vi "final.vi"() -> ()   [LabVIEW 2018]
uses:
  <vilib>/DAQmx/read.llb/DAQmx Read (Analog DBL 1Chan 1Samp).vi
  <vilib>/DAQmx/create/channels.llb/DAQmx Create Channel (AI-Voltage-Basic).vi
  <vilib>/DAQmx/miscellaneous.llb/DAQmx Fill In Error Info.vi
  <vilib>/Utility/file.llb/Write Delimited Spreadsheet (DBL).vi
  <vilib>/Waveform/WDTOps.llb/WDT Waveform to XY Pairs DBL.vi
  <instrlib>/Agilent 34405/Agilent 34405.lvlib
panel:
  in  "VISA":refnum<visa-resource-name>
  out "Voltage versus Time":dbl(graph)
  out "Current Versus time":dbl(graph)
  out "PWM Graph":waveform(dbl)(graph)
  in  "stop":bool
  in  "file path (dialog if empty)":path
  in  "Ahmeter":refnum<visa-resource-name>
  in  "Counter-clockwise":bool
  in  "Clockwise Rotation":bool
  in  "Nucleo":refnum<visa-resource-name>
  in  "Motor speed (In duty cycle %)":u8(knob) max=100 scale=0.0..100.0
  # "Probe Attenuation MUST BE SET TO X10"
  # "Notes on Controling the direction:\n\nLeaving both buttons off will set the motor to coast\nOnly turning clockwise on will set the motor to turn clockwise\nOnly turning counter-clockwise on will set the motor to turn counter clock-wise\nTurning both on will set the motor to BREAK"
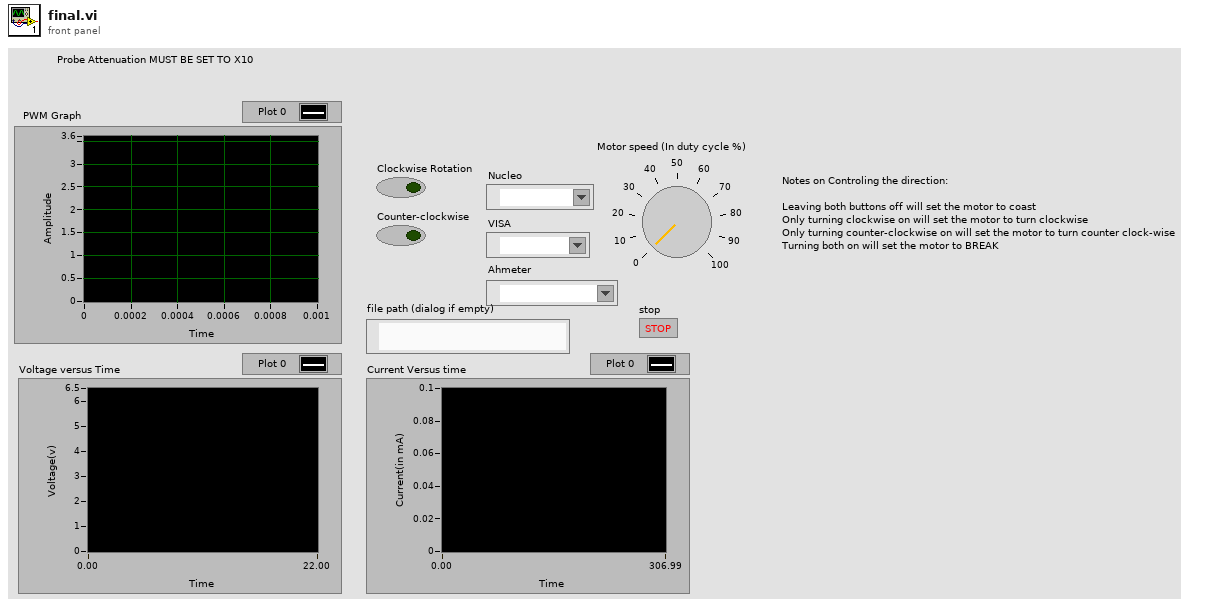
[diagram p1: front panel]
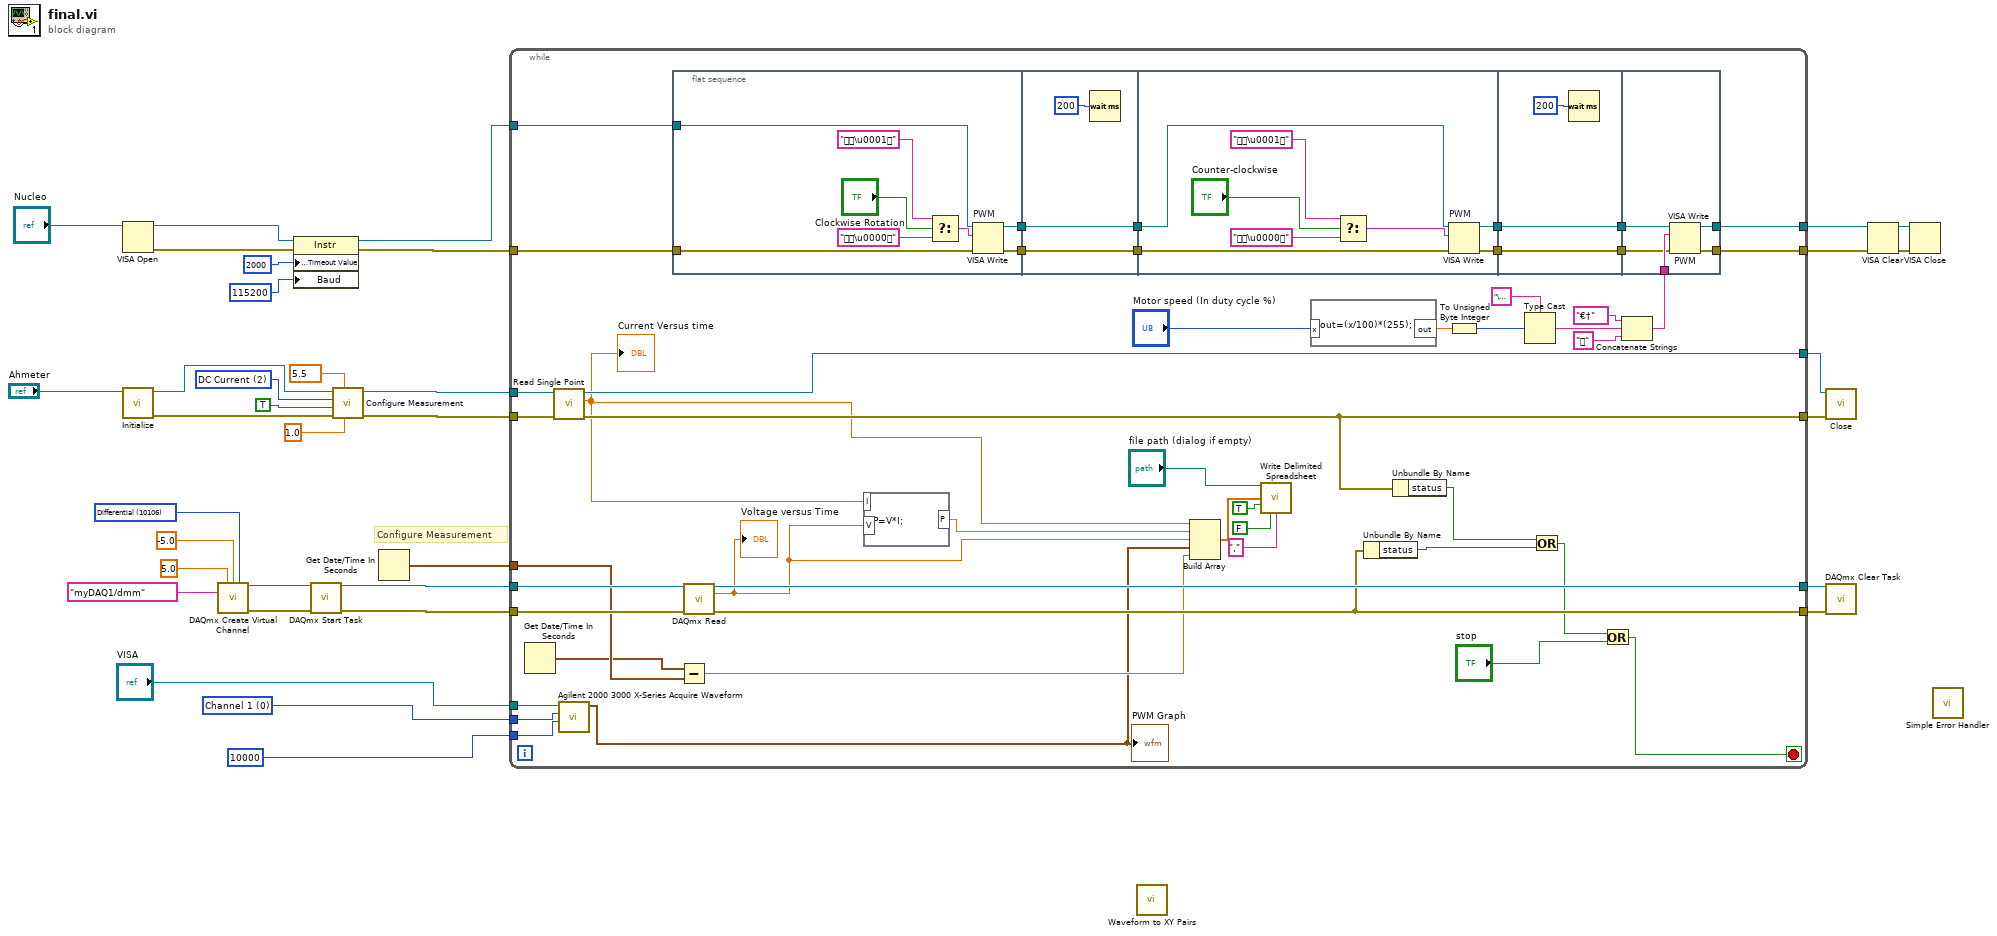
[diagram p0: block diagram]
diagram:
  w2 = 0 items=["Channel 1"=0, "Channel 2"=1, "Channel 3"=2, "Channel 4"=3, "Digital Bus Low"=9, "Digital Bus High"=10] ("Auto Scale Source (0: Channel 1)")
  w11 = 5.5 items=["3.5"=3.5, "4.5"=4.5, "5.5"=5.5] ("Manual Resolution (5.5 Digits)")
  w9 = 2 items=["DC Volts", "AC Volts", "DC Current", "AC Current", "2-Wire Resistance", "Frequency", "Temperature", "Capacitance", "Continuity", "Diode", "4-Wire Resistance", "2nd DC Volts", "2nd AC Volts", "2nd DC Current", "2nd AC Current", "2nd Frequency"] ("Function (0: DC Volts)")
  w22 = 10106 items=["Default"=-1, "RSE"=10083, "NRSE"=10078, "Differential"=10106, "Pseudodifferential"=12529] ("input terminal configuration")
  # "Configure Measurement"
  n1 = VISA Open(VISA resource name="Nucleo") -> (VISA resource name=w33:refnum<visa-resource-name>, error out=w36:errorcluster)  [unwired: 4 in]
  n2 = call <instrlib>:"Initialize.vi"("VISA resource name"="Ahmeter") -> ("error out"=w13:errorcluster, "VISA resource name out"=w14:refnum<visa-resource-name>)  [unwired: 3 in, 6 out]
  n3 = call-poly <vilib>:"DAQmx Create Virtual Channel.vi"("maximum value"=5.0, "minimum value"=-5.0, "input terminal configuration"=w22, "physical channels"=tag "myDAQ1/dmm") -> ("task out"=w27:refnum<k21>, "error out"=w26:errorcluster)  [unwired: 10 in]
  n4 = property class="Instr"(reference=w33, error in=w36, "General Settings:Timeout Value"=u32 2000, "Baud"=u32 115200 ("Serial Settings:Baud Rate")) -> (reference out=w29:refnum<visa-resource-name>, error out=w28:errorcluster)
  n5 = call <vilib>:"DAQmx Start Task.vi"("task/channels in"=w27, "error in"=w26) -> ("task out"=w19:refnum<k21>, "error out"=w18:errorcluster)  [unwired: 12 in]
  n6 = call <instrlib>:"Configure Measurement.vi"("Manual Range (1)"=1.0, "Manual Resolution (5.5 Digits)"=w11, "error in (no error)"=w13, "Enable Auto Range (T:Enable)"=TRUE, "Function (0: DC Volts)"=w9, "VISA resource name"=w14) -> ("error out"=w8:errorcluster, "VISA resource name out"=w7:refnum<visa-resource-name>)  [unwired: 4 out]
  n7 = Get Date/Time In Seconds() -> (seconds since 1Jan1904=w4:timestamp)
  n8 = while {
    tunnel: w29 -> [w84]
    tunnel: w28 -> [w83]
    tunnel: [w56] -> w21
    tunnel: [w50] -> w20
    tunnel: w19 -> [w63]
    tunnel: w18 -> [w62]
    tunnel: [w70] -> w17
    tunnel: [w69] -> w16
    tunnel: w8 -> [w68]
    tunnel: w7 -> [w67]
    tunnel: [w52] -> w6
    tunnel: [w66] -> w5
    tunnel: w4 -> [w53]
    tunnel: "VISA" -> [w40]
    tunnel: w2 -> [w39]
    tunnel: u32 10000 ("Maximum Time (10000 ms)") -> [w38]
    stop <- w46 stop-if-true
    n9 = Get Date/Time In Seconds() -> (seconds since 1Jan1904=w45:timestamp)
    n10 = call <instrlib>:"Read Single Point.vi"("error in (no error)"=w68, "VISA resource name"=w67) -> ("error out"=w52:errorcluster, "Measurement"=w42:dbl, "VISA resource name out"=w66:refnum<visa-resource-name>)  [unwired: 7 out]
    "Current Versus time" <- w42
    n11 = call "Agilent 2000 3000 X-Series Acquire Waveform.vi"("Maximum Time (10000 ms)"=w38, "Auto Scale Source (0: Channel 1)"=w39, "VISA resource name"=w40) -> ("Waveform Data"=w37:waveform(dbl))  [unwired: 8 in]
    "PWM Graph" <- w37
    n12 = flat-sequence {
      tunnel: [w90] -> w78
      tunnel: [w89] -> w77
      tunnel: w84 -> [w92]
      tunnel: w83 -> [w91]
      tunnel: w78 -> [w95]
      tunnel: w77 -> [w94]
      tunnel: [w95] -> w76
      tunnel: [w94] -> w75
      tunnel: w76 -> [w98]
      tunnel: w75 -> [w99]
      tunnel: [w97] -> w65
      tunnel: [w96] -> w64
      tunnel: w65 -> [w104]
      tunnel: w64 -> [w105]
      tunnel: [w105] -> w61
      tunnel: [w104] -> w60
      tunnel: w71 -> [w111]
      tunnel: [w110] -> w70
      tunnel: [w109] -> w69
      tunnel: w61 -> [w108]
      tunnel: w60 -> [w107]
      frame #0 {
        n13 = Select(t="\u0001" ("write buffer"), s="Clockwise Rotation", f="\u0000" ("write buffer")) -> (s? t:f=w85:string)
        n14 = VISA Write "PWM"(VISA resource name=w92, write buffer=w85, error in (no error)=w91) -> (VISA resource name out=w90:refnum<visa-resource-name>, error out=w89:errorcluster)  [unwired: 1 out]
      }
      frame #1 {
        n15 = Wait (ms)(milliseconds to wait=u32 200) -> ()  [unwired: 1 out]
      }
      frame #2 {
        n16 = Select(t="\u0001" ("write buffer"), s="Counter-clockwise", f="\u0000" ("write buffer")) -> (s? t:f=w103:string)
        n17 = VISA Write "PWM"(VISA resource name=w98, write buffer=w103, error in (no error)=w99) -> (VISA resource name out=w96:refnum<visa-resource-name>, error out=w97:errorcluster)  [unwired: 1 out]
      }
      frame #3 {
        n18 = Wait (ms)(milliseconds to wait=u32 200) -> ()  [unwired: 1 out]
      }
      frame #4 {
        n19 = VISA Write "PWM"(VISA resource name=w108, write buffer=w111, error in (no error)=w107) -> (VISA resource name out=w110:refnum<visa-resource-name>, error out=w109:errorcluster)  [unwired: 1 out]
      }
    }
    n20 = Subtract(x=w45, y=w53) -> (x-y=w43:dbl)
    n21 = call-poly <vilib>:"DAQmx Read.vi"("task/channels in"=w63, "error in"=w62) -> ("task out"=w56:refnum<k21>, "data"=w41:dbl, "error out"=w50:errorcluster)  [unwired: 11 in]
    "Voltage versus Time" <- w41
    n22 = formula code="P=V*I;"("V"=w41, "I"=w42) -> ("P"=w44:dbl)
    n23 = Build Array(w42, w44, w41, w37, w43) -> (w55:dbl[])
    n24 = call-poly <vilib>:"Write Delimited Spreadsheet.vi"("file path (dialog if empty)"="file path (dialog if empty)", "1D data"=w55, "append to file? (new file:F)"=TRUE, "transpose? (no:F)"=FALSE, "delimiter (\\t)"="," ("delimiter (\\t)")) -> ()  [unwired: 9 in, 2 out]
    n25 = formula code="out=(x/100)*(255);"("x"="Motor speed (In duty cycle %)") -> ("out"=w82:dbl)
    n26 = Unbundle By Name(w50) -> ("status"=w49:bool)
    n27 = Unbundle By Name(w52) -> ("status"=w51:bool)
    n28 = To Unsigned Byte Integer(number=w82) -> (unsigned 8bit integer=w81:u8)
    n29 = Type Cast(type="\u0000", x=w81) -> (*(type *) &x=w73:string)
    n30 = Or(x=w51, y=w49) -> (x .or. y?=w48:bool)
    n31 = Or(x=w48, y="stop") -> (x .or. y?=w46:bool)
    n32 = Concatenate Strings("€†" ("string"), w73, "" ("string")) -> (w71:string)
  }
  n33 = call-poly <vilib>:"Waveform to XY Pairs.vi"() -> ()  [unwired: 9 in, 3 out]
  n34 = call <instrlib>:"Close.vi"("error in (no error)"=w6, "VISA resource name"=w5) -> ()  [unwired: 10 out]
  n35 = call <vilib>:"DAQmx Clear Task.vi"("task in"=w21, "error in"=w20) -> ()  [unwired: 13 in, 1 out]
  n36 = VISA Clear(VISA resource name=w17, error in (no error)=w16) -> (VISA resource name out=w30:refnum<visa-resource-name>, error out=w31:errorcluster)
  n37 = VISA Close(VISA resource name=w30, error in (no error)=w31) -> ()  [unwired: 1 out]
  n38 = call <vilib>:"Simple Error Handler.vi"() -> ()  [unwired: 2 in, 8 out]
